vi "电机控制.vi"() -> ()   [LabVIEW 2016]
uses:
  <vilib>/Instr/_visa.llb/VISA Configure Serial Port (Instr).vi
panel:
  in  "选项卡控件":T1
  in  "PID_控制\n方式切换":bool
  in  "复位":bool
  in  "启动电机":bool
  in  "PID":cluster{"P":sgl, "I":sgl, "D":sgl} {"D" min=0 max=100 step=0.1 format="%.1f"; "I" min=0 max=100 step=0.1 format="%.1f"; "P" min=0 max=100 step=0.1 format="%.1f"}
  in  "发送目标值":bool
  in  "目标值":u32
  in  "发送PID":bool
  out "波形图表":cluster{"实际值 ":u32, "目标值":u32}(graph)
  out "串口指示灯":bool
  in  "确定按钮":bool
  in  "串口配置簇":T2={"端口"="", "波特率"=115200, "数据位"=8, "停止位"=10, "校验位"=0} {"校验位" items=["无", "奇校验", "偶校验", "Mark", "Space"]; "停止位" items=["1"=10, "2"=20]; "数据位" items=["5"=5, "6"=6, "7"=7, "8"=8]; "波特率" items=["4800"=4800, "9600"=9600, "57600"=57600, "115200"=115200]}
  out "电机转速":u32
  out "控制模\n式显示":string
  out "转速表":u32(knob) scale=0.0..230.0
  in  "转盘":u32(knob) caption="角度控制" max=360 step=20 scale=0.0..360.0
  in  "速度控制":u32(knob) max=210 step=1 scale=0.0..210.0
  out "波形图表":dbl(graph)
  out "位置控制\nPID参数":sgl[](array[numeric])
  out "速度控制\nPID":sgl[](array[numeric])
  out "指令":string
  out "16进制字符串":string
  out "接收字节数":u32
  out "error out":errorcluster
  # "电机控制调试助手"
  # "PID配置"
  # "串口配置"
  # "操作"
  # "r/min"
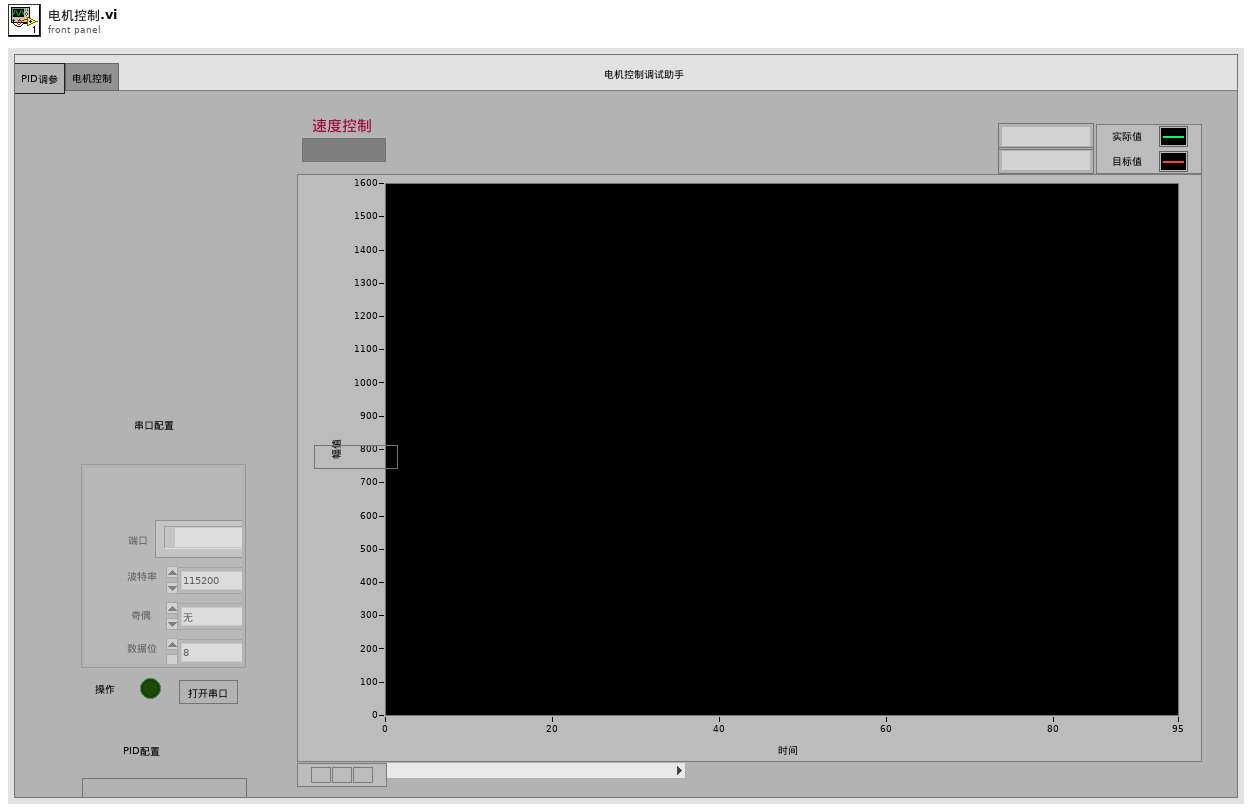
[diagram p1: front panel]
types:
  T1 = typedef "控件 2.ctl" = enum32{"PID调参", "电机控制"}
  T2 = cluster{"端口":refnum<visa-resource-name>, "波特率":u32, "数据位":u16, "停止位":u16, "校验位":u16}
  T3 = enum8{"Enabled", "Disabled", "Disabled and Grayed Out"}
  T4 = cluster{"PID[0]":sgl, "PID[1]":sgl, "PID[2]":sgl}
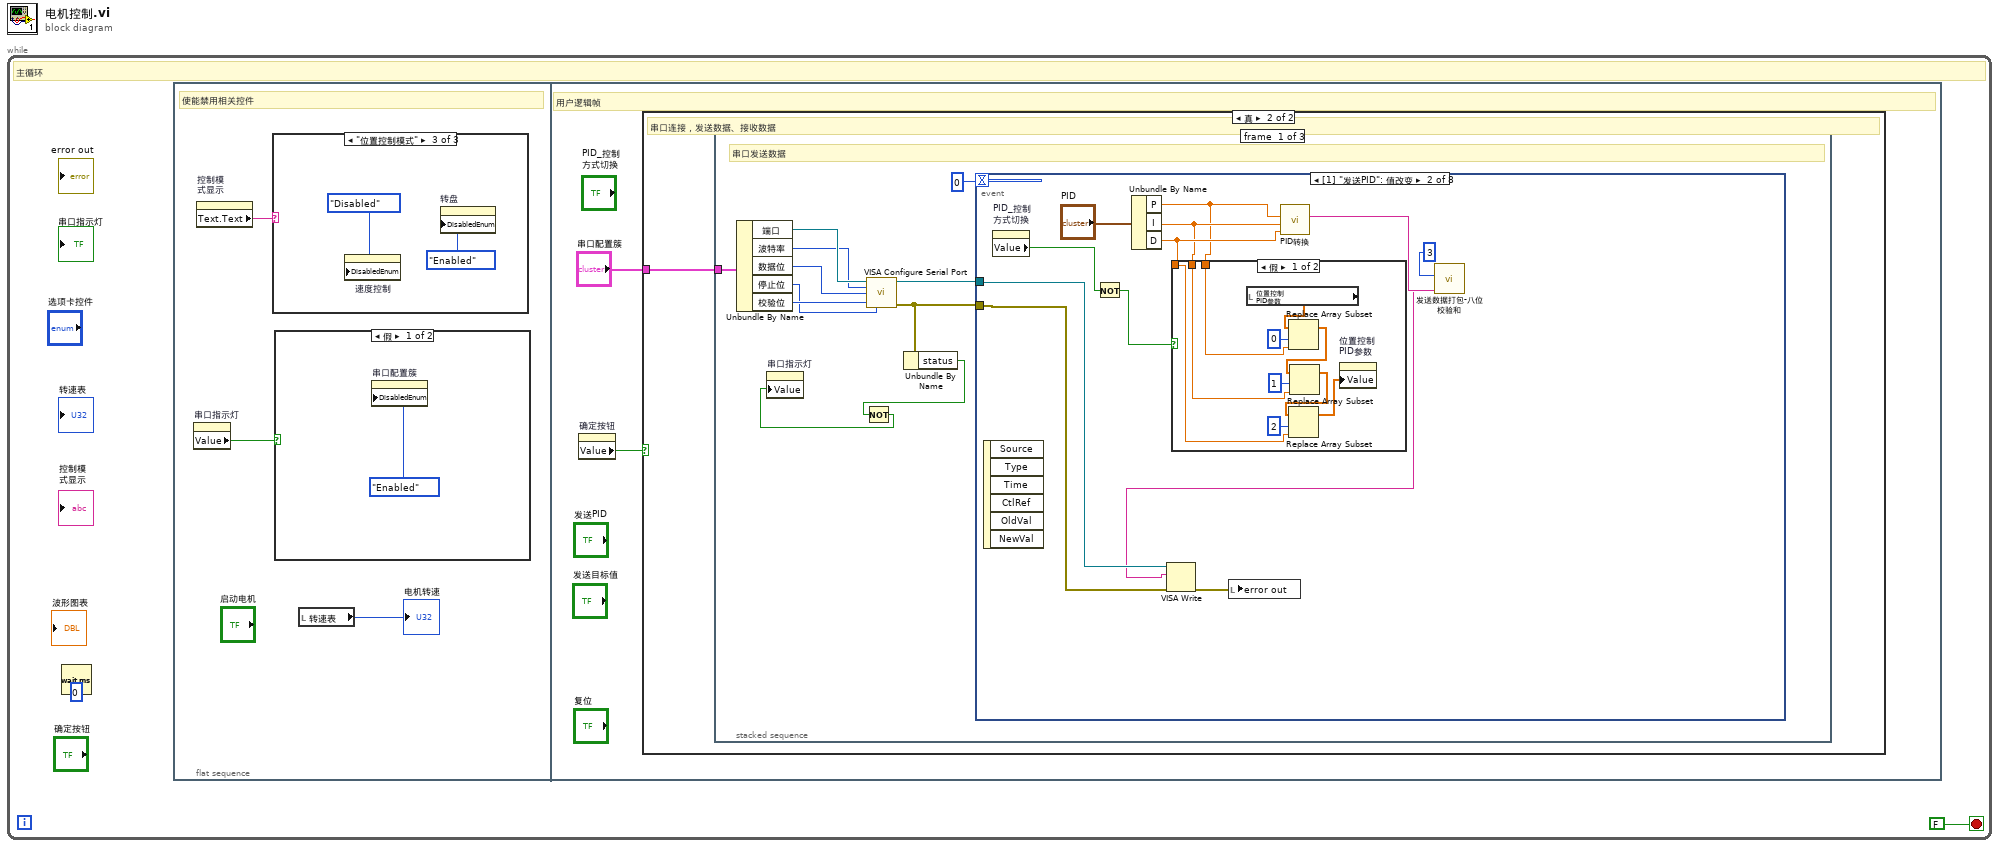
[diagram p0: block diagram]
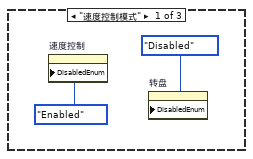
[diagram p2: hidden frame]
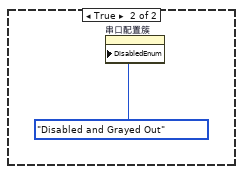
[diagram p4: hidden frame]
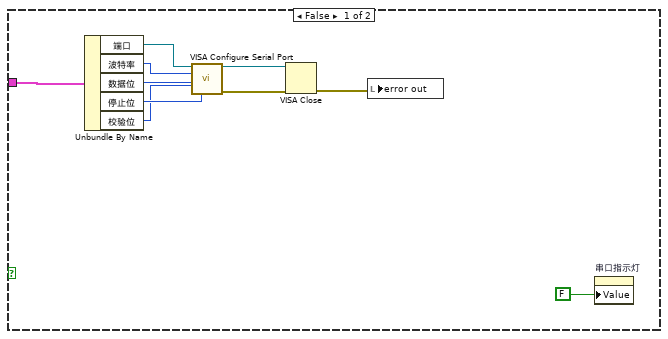
[diagram p5: hidden frame]
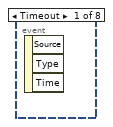
[diagram p6: hidden frame]
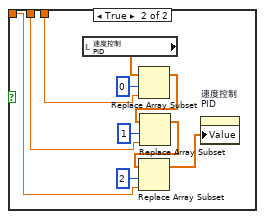
[diagram p7: hidden frame]
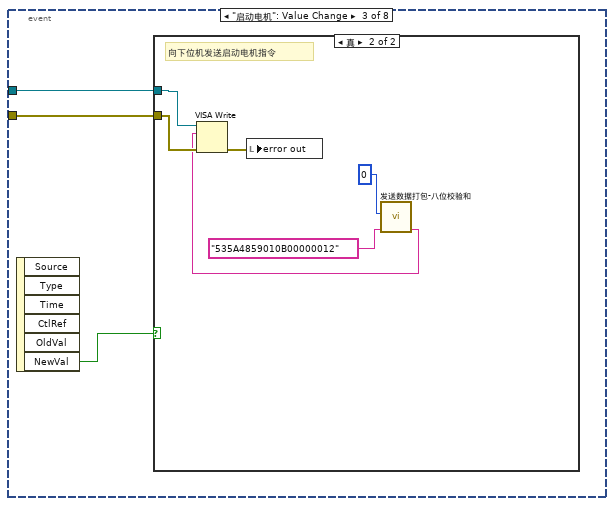
[diagram p8: hidden frame]
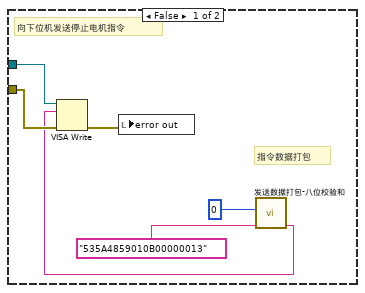
[diagram p9: hidden frame]
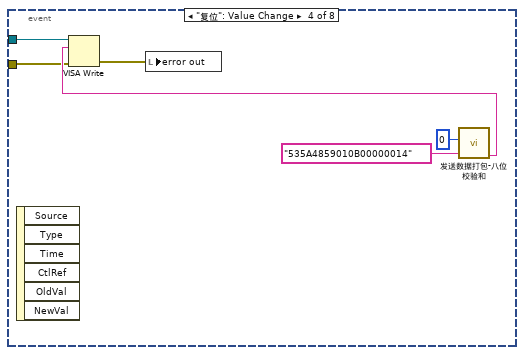
[diagram p10: hidden frame]
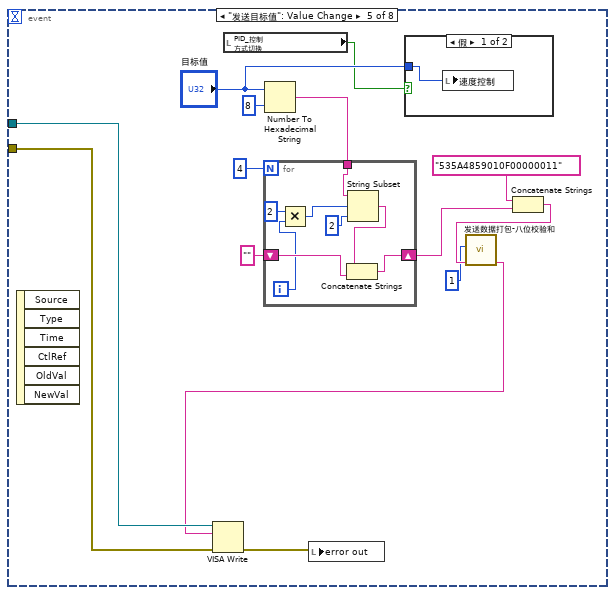
[diagram p11: hidden frame]
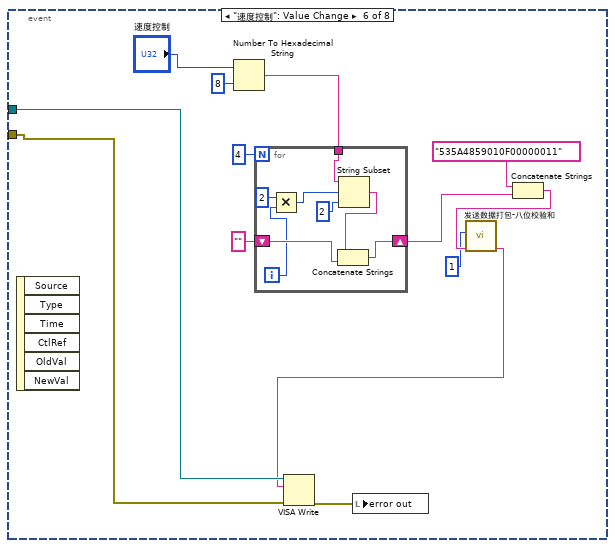
[diagram p13: hidden frame]
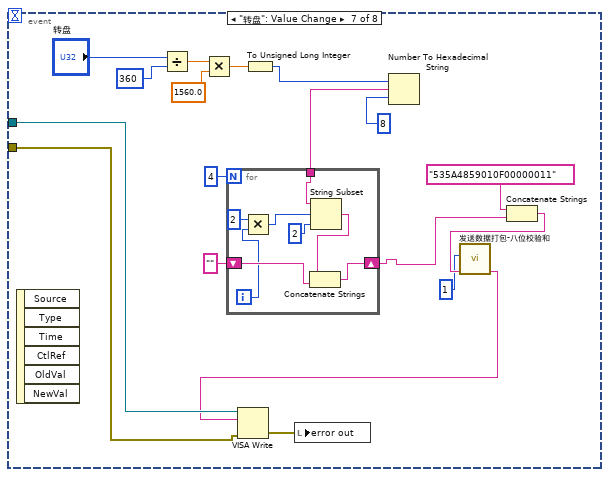
[diagram p14: hidden frame]
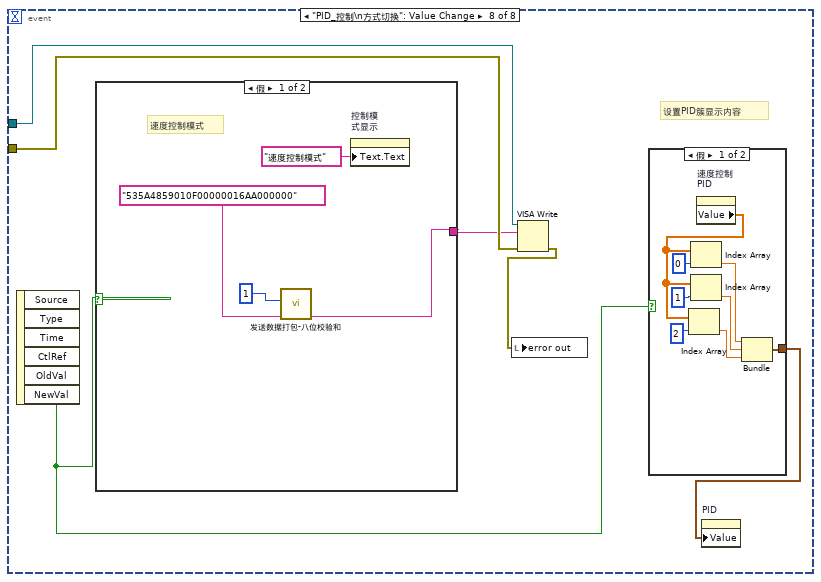
[diagram p15: hidden frame]
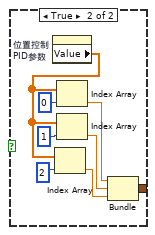
[diagram p16: hidden frame]
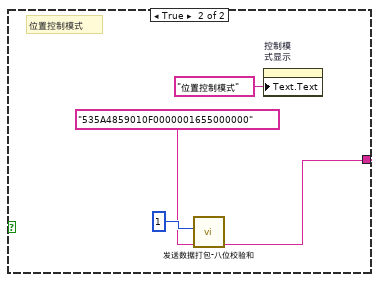
[diagram p17: hidden frame]
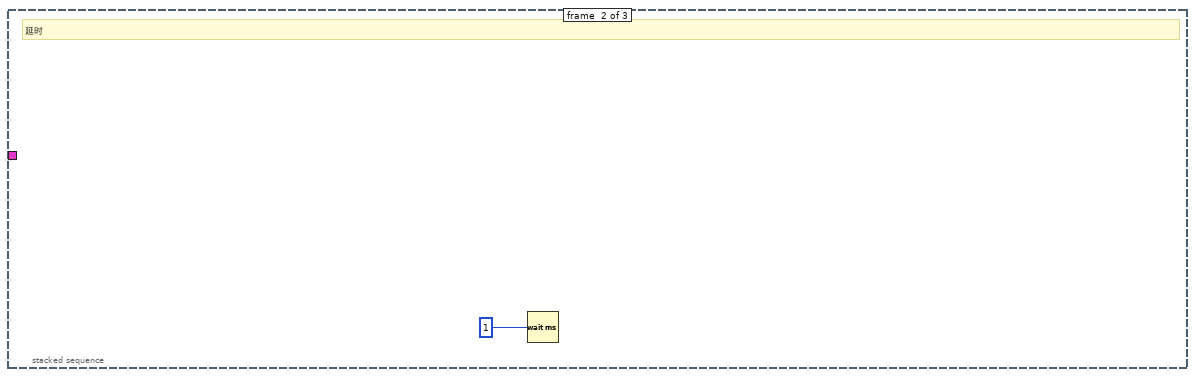
[diagram p18: hidden frame]
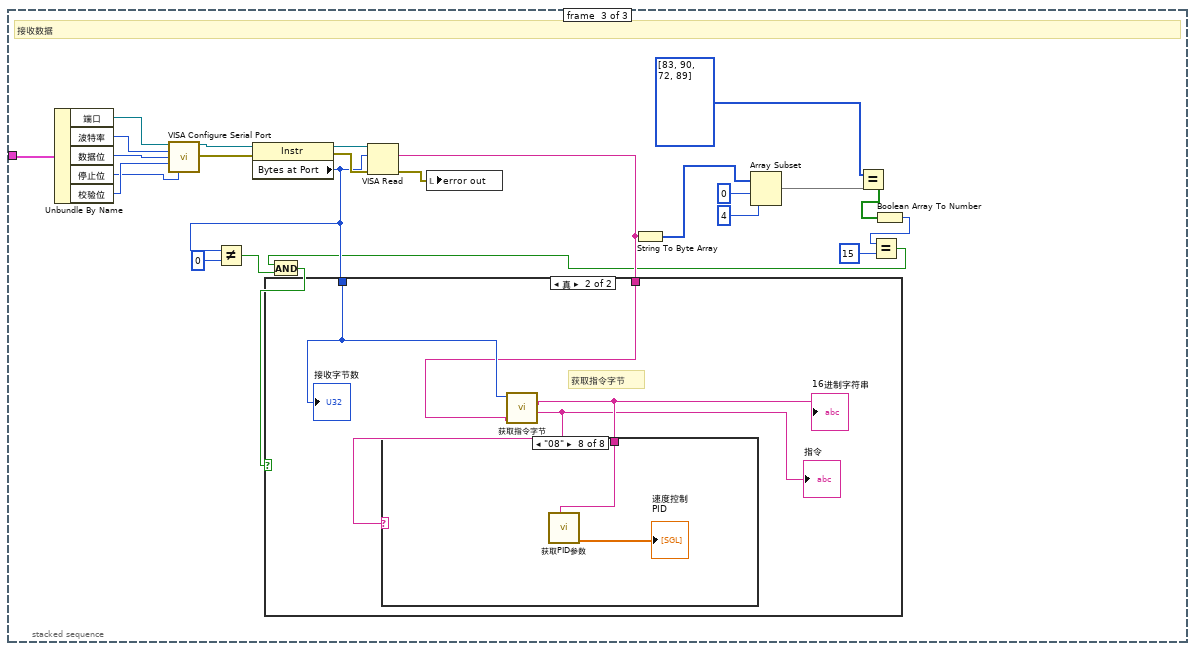
[diagram p19: hidden frame]
diagram:
  n1 = while {
    stop <- FALSE stop-if-true
    # "主循环"
    n2 = Wait (ms)(milliseconds to wait=u32 0 ("等待时间（毫秒）")) -> ()  [unwired: 1 out]
    n3 = flat-sequence {
      frame #0 {
        # "使能禁用相关控件"
        n4 = property on="串口指示灯" class="Bool (严格)"() -> ("Value"=w5:bool)  [unwired: 2 in, 2 out]
        n5 = property on="控制模\n式显示" class="Str"() -> ("Text.Text"=w3:string)  [unwired: 2 in, 2 out]
        n6 = case shown="\"位置控制模式\"" w3 {
          frame "速度控制模式" {
            n7 = property on="速度控制" class="Knob (严格)"("DisabledEnum"=T3."Enabled" ("禁用")) -> ()  [unwired: 2 in, 2 out]
            n8 = property on="转盘" class="Knob (严格)"("DisabledEnum"=T3."Disabled" ("禁用")) -> ()  [unwired: 2 in, 2 out]
          }
          frame "假", Default {
          }
          frame "位置控制模式" {
            n9 = property on="速度控制" class="Knob (严格)"("DisabledEnum"=T3."Disabled" ("禁用")) -> ()  [unwired: 2 in, 2 out]
            n10 = property on="转盘" class="Knob (严格)"("DisabledEnum"=T3."Enabled" ("禁用")) -> ()  [unwired: 2 in, 2 out]
          }
        }
        n11 = case shown="假" w5 {
          frame False {
            n12 = property on="串口配置簇" class="Clust (严格)"("DisabledEnum"=T3."Enabled" ("禁用")) -> ()  [unwired: 2 in, 2 out]
          }
          frame True {
            n13 = property on="串口配置簇" class="Clust (严格)"("DisabledEnum"=T3."Disabled and Grayed Out" ("禁用")) -> ()  [unwired: 2 in, 2 out]
          }
        }
        n14 = local read "转速表"() -> (→"电机转速":u32)
      }
      frame #1 {
        # "用户逻辑帧"
        n15 = property on="确定按钮" class="Bool (严格)"() -> ("Value"=w13:bool)  [unwired: 2 in, 2 out]
        n16 = case shown="真" w13 {
          tunnel: "串口配置簇" -> [w22 w24]
          frame False {
            n17 = Unbundle By Name(w22) -> ("端口"=w21:refnum<visa-resource-name>, "波特率"=w20:u32, "数据位"=w19:u16, "停止位"=w18:u16, "校验位"=w17:u16)
            n18 = call-poly "VISA Configure Serial Port"("VISA resource name"=w21, "baud rate (9600)"=w20, "data bits (8)"=w19, "parity (0:none)"=w17, "stop bits (10: 1 bit)"=w18) -> ("VISA resource name out"=w16:refnum<visa-resource-name>, "error out"=w15:errorcluster)  [unwired: 9 in]
            n19 = VISA Close(VISA resource name=w16, error in (no error)=w15) -> (error out=w14:errorcluster)
            n20 = local write "error out"(w14) -> ()
            n21 = property on="串口指示灯" class="Bool (严格)"("Value"=FALSE ("串口指示灯")) -> ()  [unwired: 2 in, 2 out]
          }
          frame True {
            # "串口连接，发送数据、接收数据"
            n22 = stacked-sequence {
              tunnel: w24 -> [w33 _ w214]
              frame #0 {
                # "串口发送数据"
                n23 = Unbundle By Name(w33) -> ("端口"=w32:refnum<visa-resource-name>, "波特率"=w31:u32, "数据位"=w30:u16, "停止位"=w28:u16, "校验位"=w29:u16)
                n24 = call-poly "VISA Configure Serial Port"("VISA resource name"=w32, "baud rate (9600)"=w31, "data bits (8)"=w30, "parity (0:none)"=w29, "stop bits (10: 1 bit)"=w28) -> ("VISA resource name out"=w34:refnum<visa-resource-name>, "error out"=w25:errorcluster)  [unwired: 9 in]
                n25 = Unbundle By Name(w25) -> ("status"=w27:bool)
                n26 = Not(x=w27) -> (.not. x?=w26:bool)
                n27 = property on="串口指示灯" class="Bool (严格)"("Value"=w26) -> ()  [unwired: 2 in, 2 out]
                n28 = event shown="[1] \"发送PID\": 值改变" {
                  selector: _ -> [_ _ _ _ _ _ _ _]
                  dyn-events: _ -> [_ _ _ _ _ _ _ _]
                  timeout: 0 -> [_ _ _ _ _ _ _ _]
                  tunnel: w34 -> [_ w47 w69 w84 w102 w116 w142 w164]
                  tunnel: w25 -> [_ w46 w68 w85 w101 w115 w141 w163]
                  event Timeout {
                    n29 = event-data() -> ()  [unwired: 1 in, 3 out]
                  }
                  event "发送PID": Value Change {
                    n30 = event-data() -> ()  [unwired: 1 in, 6 out]
                    n31 = property on="PID_控制\n方式切换" class="Bool (严格)"() -> ("Value"=w37:bool)  [unwired: 2 in, 2 out]
                    n32 = Not(x=w37) -> (.not. x?=w36:bool)
                    n33 = Unbundle By Name("PID") -> ("P"=w38:sgl, "I"=w39:sgl, "D"=w40:sgl)
                    n34 = case shown="假" w36 {
                      tunnel: w40 -> [w48 w59]
                      tunnel: w39 -> [w49 w60]
                      tunnel: w38 -> [w50 w61]
                      frame False {
                        n35 = local read "位置控制\nPID参数"() -> (w52:sgl[])
                        n36 = Replace Array Subset(array=w52, new element=w50, index=0 ("索引")) -> (w54:sgl[])
                        n37 = Replace Array Subset(array=w54, new element=w49, index=1 ("索引")) -> (w53:sgl[])
                        n38 = Replace Array Subset(array=w53, new element=w48, index=2 ("索引")) -> (w51:sgl[])
                        n39 = property on="位置控制\nPID参数" class="Arr (严格)"("Value"=w51) -> ()  [unwired: 2 in, 2 out]
                      }
                      frame True {
                        n40 = local read "速度控制\nPID"() -> (w67:sgl[])
                        n41 = Replace Array Subset(array=w67, new element=w61, index=0 ("索引")) -> (w66:sgl[])
                        n42 = Replace Array Subset(array=w66, new element=w60, index=1 ("索引")) -> (w65:sgl[])
                        n43 = Replace Array Subset(array=w65, new element=w59, index=2 ("索引")) -> (w58:sgl[])
                        n44 = property on="速度控制\nPID" class="Arr (严格)"("Value"=w58) -> ()  [unwired: 2 in, 2 out]
                      }
                    }
                    n45 = call "PID转换.vi"("P"=w38, "I"=w39, "D"=w40) -> ("PID"=w43:string)  [unwired: 7 in]
                    n46 = call "发送数据打包-八位校验和.vi"("16进制字符串"=w43, "命令数"=u8 3) -> ("结果字符串"=w42:string)  [unwired: 8 in, 1 out]
                    n47 = VISA Write(VISA resource name=w47, write buffer=w42, error in (no error)=w46) -> (error out=w45:errorcluster)  [unwired: 2 out]
                    n48 = local write "error out"(w45) -> ()
                  }
                  event "启动电机": Value Change {
                    n49 = event-data() -> ("NewVal"=w70:bool)  [unwired: 1 in, 5 out]
                    n50 = case shown="真" w70 {
                      tunnel: w69 -> [w73 w81]
                      tunnel: w68 -> [w72 w82]
                      frame False {
                        # "指令数据打包"
                        # "向下位机发送停止电机指令"
                        n51 = call "发送数据打包-八位校验和.vi"("16进制字符串"="535A4859010B00000013", "命令数"=u8 0) -> ("结果字符串"=w71:string)  [unwired: 8 in, 1 out]
                        n52 = VISA Write(VISA resource name=w73, write buffer=w71, error in (no error)=w72) -> (error out=w76:errorcluster)  [unwired: 2 out]
                        n53 = local write "error out"(w76) -> ()
                      }
                      frame True {
                        # "向下位机发送启动电机指令"
                        n54 = call "发送数据打包-八位校验和.vi"("16进制字符串"="535A4859010B00000012", "命令数"=u8 0) -> ("结果字符串"=w77:string)  [unwired: 8 in, 1 out]
                        n55 = VISA Write(VISA resource name=w81, write buffer=w77, error in (no error)=w82) -> (error out=w80:errorcluster)  [unwired: 2 out]
                        n56 = local write "error out"(w80) -> ()
                      }
                    }
                  }
                  event "复位": Value Change {
                    n57 = event-data() -> ()  [unwired: 1 in, 6 out]
                    n58 = call "发送数据打包-八位校验和.vi"("16进制字符串"="535A4859010B00000014", "命令数"=u8 0) -> ("结果字符串"=w86:string)  [unwired: 8 in, 1 out]
                    n59 = VISA Write(VISA resource name=w84, write buffer=w86, error in (no error)=w85) -> (error out=w83:errorcluster)  [unwired: 2 out]
                    n60 = local write "error out"(w83) -> ()
                  }
                  event "发送目标值": Value Change {
                    n61 = event-data() -> ()  [unwired: 1 in, 6 out]
                    n62 = local read "PID_控制\n方式切换"() -> (w89:bool)
                    n63 = Number To Hexadecimal String(1:i16 8 ("宽度(-)"), 2:"目标值") -> (0:w98:string)
                    n64 = for {
                      N: 4 -> [_]
                      tunnel: w98 -> [w111]
                      shift-right: [w109] -> w94
                      shift-left: "" -> [w108]
                      i -> [w106]
                      n65 = Multiply(x=2, y=w106) -> (x*y=w104:i32)
                      n66 = String Subset(string=w111, offset (0)=w104, length (rest)=u8 2 ("y")) -> (substring=w107:string)
                      n67 = Concatenate Strings(w107, w108) -> (w109:string)
                    }
                    n68 = case shown="假" w89 {
                      tunnel: "目标值" -> [w103 _]
                      frame False {
                        n69 = local write "速度控制"(w103) -> ()
                      }
                      frame True {
                      }
                    }
                    n70 = Concatenate Strings("535A4859010F00000011", w94) -> (w93:string)
                    n71 = call "发送数据打包-八位校验和.vi"("16进制字符串"=w93, "命令数"=u8 1) -> ("结果字符串"=w91:string)  [unwired: 8 in, 1 out]
                    n72 = VISA Write(VISA resource name=w102, write buffer=w91, error in (no error)=w101) -> (error out=w100:errorcluster)  [unwired: 2 out]
                    n73 = local write "error out"(w100) -> ()
                  }
                  event "速度控制": Value Change {
                    n74 = event-data() -> ()  [unwired: 1 in, 6 out]
                    n75 = Number To Hexadecimal String(1:i16 8 ("宽度(-)"), 2:"速度控制") -> (0:w123:string)
                    n76 = for {
                      N: 4 -> [_]
                      tunnel: w123 -> [w132]
                      shift-right: [w130] -> w119
                      shift-left: "" -> [w129]
                      i -> [w127]
                      n77 = Multiply(x=2, y=w127) -> (x*y=w125:i32)
                      n78 = String Subset(string=w132, offset (0)=w125, length (rest)=u8 2 ("y")) -> (substring=w128:string)
                      n79 = Concatenate Strings(w128, w129) -> (w130:string)
                    }
                    n80 = Concatenate Strings("535A4859010F00000011", w119) -> (w121:string)
                    n81 = call "发送数据打包-八位校验和.vi"("16进制字符串"=w121, "命令数"=u8 1) -> ("结果字符串"=w113:string)  [unwired: 8 in, 1 out]
                    n82 = VISA Write(VISA resource name=w116, write buffer=w113, error in (no error)=w115) -> (error out=w114:errorcluster)  [unwired: 2 out]
                    n83 = local write "error out"(w114) -> ()
                  }
                  event "转盘": Value Change {
                    n84 = event-data() -> ()  [unwired: 1 in, 6 out]
                    n85 = Divide(x="转盘", y=u32 360) -> (x/y=w136:dbl)
                    n86 = Multiply(x=w136, y=1560.0) -> (x*y=w134:dbl)
                    n87 = To Unsigned Long Integer(number=w134) -> (unsigned 32bit integer=w133:u32)
                    n88 = Number To Hexadecimal String(1:i16 8 ("宽度(-)"), 2:w133) -> (0:w149:string)
                    n89 = for {
                      N: 4 -> [_]
                      tunnel: w149 -> [w158]
                      shift-right: [w156] -> w143
                      shift-left: "" -> [w155]
                      i -> [w153]
                      n90 = Multiply(x=2, y=w153) -> (x*y=w151:i32)
                      n91 = String Subset(string=w158, offset (0)=w151, length (rest)=u8 2 ("y")) -> (substring=w154:string)
                      n92 = Concatenate Strings(w154, w155) -> (w156:string)
                    }
                    n93 = Concatenate Strings("535A4859010F00000011", w143) -> (w145:string)
                    n94 = call "发送数据打包-八位校验和.vi"("16进制字符串"=w145, "命令数"=u8 1) -> ("结果字符串"=w139:string)  [unwired: 8 in, 1 out]
                    n95 = VISA Write(VISA resource name=w142, write buffer=w139, error in (no error)=w141) -> (error out=w140:errorcluster)  [unwired: 2 out]
                    n96 = local write "error out"(w140) -> ()
                  }
                  event "PID_控制\n方式切换": Value Change {
                    # "设置PID簇显示内容"
                    n97 = event-data() -> ("NewVal"=w159:bool)  [unwired: 1 in, 5 out]
                    n98 = case shown="假" w159 {
                      tunnel: [w182 w186] -> w162
                      frame False {
                        # "速度控制模式"
                        n99 = call "发送数据打包-八位校验和.vi"("16进制字符串"="535A4859010F00000016AA000000", "命令数"=u8 1) -> ("结果字符串"=w182:string)  [unwired: 8 in, 1 out]
                        n100 = property on="控制模\n式显示" class="Str"("Text.Text"="速度控制模式" ("文本.文本")) -> ()  [unwired: 2 in, 2 out]
                      }
                      frame True {
                        # "位置控制模式"
                        n101 = call "发送数据打包-八位校验和.vi"("16进制字符串"="535A4859010F0000001655000000", "命令数"=u8 1) -> ("结果字符串"=w186:string)  [unwired: 8 in, 1 out]
                        n102 = property on="控制模\n式显示" class="Str"("Text.Text"="位置控制模式" ("文本.文本")) -> ()  [unwired: 2 in, 2 out]
                      }
                    }
                    n103 = VISA Write(VISA resource name=w164, write buffer=w162, error in (no error)=w163) -> (error out=w161:errorcluster)  [unwired: 2 out]
                    n104 = local write "error out"(w161) -> ()
                    n105 = case shown="假" w159 {
                      tunnel: [w165 w173] -> w160
                      frame False {
                        n106 = property on="速度控制\nPID" class="Arr (严格)"() -> ("Value"=w166:sgl[])  [unwired: 2 in, 2 out]
                        n107 = Index Array(array=w166, index=2 ("索引")) -> (element=w167:sgl)
                        n108 = Index Array(array=w166, index=0 ("索引")) -> (element=w170:sgl)
                        n109 = Index Array(array=w166, index=1 ("索引")) -> (element=w169:sgl)
                        n110 = Bundle(w170, w169, w167) -> (w165:cluster{sgl, sgl, sgl})  [unwired: 1 in]
                      }
                      frame True {
                        n111 = property on="位置控制\nPID参数" class="Arr (严格)"() -> ("Value"=w176:sgl[])  [unwired: 2 in, 2 out]
                        n112 = Index Array(array=w176, index=2 ("索引")) -> (element=w174:sgl)
                        n113 = Index Array(array=w176, index=0 ("索引")) -> (element=w178:sgl)
                        n114 = Index Array(array=w176, index=1 ("索引")) -> (element=w177:sgl)
                        n115 = Bundle(w178, w177, w174) -> (w173:cluster{sgl, sgl, sgl})  [unwired: 1 in]
                      }
                    }
                    n116 = property on="PID" class="Clust (严格)"("Value"=w160) -> ()  [unwired: 2 in, 2 out]
                  }
                }
              }
              frame #1 {
                # "延时"
                n117 = Wait (ms)(milliseconds to wait=u32 1 ("等待时间（毫秒）")) -> ()  [unwired: 1 out]
              }
              frame #2 {
                # "接收数据"
                n118 = Unbundle By Name(w214) -> ("端口"=w213:refnum<visa-resource-name>, "波特率"=w212:u32, "数据位"=w207:u16, "停止位"=w205:u16, "校验位"=w206:u16)
                n119 = call-poly "VISA Configure Serial Port"("VISA resource name"=w213, "baud rate (9600)"=w212, "data bits (8)"=w207, "parity (0:none)"=w206, "stop bits (10: 1 bit)"=w205) -> ("VISA resource name out"=w211:refnum<visa-resource-name>, "error out"=w210:errorcluster)  [unwired: 9 in]
                n120 = property class="Instr"(reference=w211, error in=w210) -> (reference out=w209:refnum<visa-resource-name>, error out=w208:errorcluster, "Bytes at Port"=w203:u32)
                n121 = Not Equal?(x=w203, y=u32 0) -> (x != y?=w193:bool)
                n122 = VISA Read(VISA resource name=w209, byte count=w203, error in (no error)=w208) -> (read buffer=w196:string, error out=w202:errorcluster)  [unwired: 2 out]
                n123 = local write "error out"(w202) -> ()
                n124 = String To Byte Array(string=w196) -> (unsigned byte array=w190:u8[])
                n125 = Array Subset(array=w190, index=0 ("索引"), length=4 ("长度")) -> (w198:u8[])
                n126 = Equal?(x=u8[] [83, 90, 72, 89], y=w198) -> (x = y?=w199:bool[])
                n127 = Boolean Array To Number(Boolean array=w199) -> (number=w195:u32)
                n128 = Equal?(x=w195, y=u32 15) -> (x = y?=w192:bool)
                n129 = And(x=w192, y=w193) -> (x .and. y?=w191:bool)
                n130 = case shown="真" w191 {
                  tunnel: w196 -> [_ w217]
                  tunnel: w203 -> [_ w218]
                  frame False {
                  }
                  frame True {
                    # "获取指令字节"
                    n131 = call "获取指令字节.vi"("字符串"=w217, "字节数"=w218) -> ("指令"=w215:string, "16进制字符串"=w216:string)  [unwired: 8 in]
                    "16进制字符串" <- w216
                    "指令" <- w215
                    n132 = case shown="\"08\"" w215 {
                      tunnel: w216 -> [_ w221 w226 w231 _ _ w237 w241]
                      frame "假", Default {
                      }
                      frame "01" {
                        n133 = call "获取实际值.vi"("字符串"=w221) -> ("实际值字符串"=w220:string)  [unwired: 9 in, 1 out]
                        n134 = Hexadecimal String To Number(string=w220) -> (number=w219:u32)  [unwired: 2 in, 1 out]
                        n135 = property on="目标值" class="DigNum (严格)"("Value"=w219) -> ()  [unwired: 2 in, 2 out]
                      }
                      frame "02" {
                        # "获取实际值"
                        # "下位机发送实际值"
                        n136 = local read "目标值"() -> (w225:u32)
                        n137 = call "获取实际值.vi"("字符串"=w226) -> ("实际值"=w222:u32)  [unwired: 9 in, 1 out]
                        n138 = local read "PID_控制\n方式切换"() -> (w223:bool)
                        n139 = Bundle("实际值"=w222, "目标值"=w225) -> (→"波形图表":cluster{"实际值 ":u32, "目标值":u32})  [unwired: 1 in]
                        n140 = case shown="假" w223 {
                          tunnel: w222 -> [w227 w228]
                          frame False {
                            n141 = local write "转速表"(w227) -> ()
                            n142 = local write "波形图表"(w227) -> ()
                          }
                          frame True {
                            n143 = local write "波形图表"(w228) -> ()
                          }
                        }
                      }
                      frame "03" {
                        # "获取PID参数"
                        n144 = call "获取PID参数.vi"("字符串"=w231) -> ("PID"=w230:sgl[])  [unwired: 10 in]
                        "位置控制\nPID参数" <- w230
                        n145 = Array To Cluster(array=w230) -> (cluster=w229:T4)
                        n146 = local write "PID"(w229) -> ()
                      }
                      frame "04" {
                        # "下位机发送启动按钮状态"
                        n147 = property on="启动电机" class="Bool (严格)"("Value"=TRUE ("启动电机")) -> ()  [unwired: 2 in, 2 out]
                      }
                      frame "05" {
                        # "下位机发送停止按钮状态"
                        n148 = property on="启动电机" class="Bool (严格)"("Value"=FALSE ("启动电机")) -> ()  [unwired: 2 in, 2 out]
                      }
                      frame "07" {
                        n149 = call "获取实际值.vi"("字符串"=w237) -> ("实际值字符串"=w236:string)  [unwired: 9 in, 1 out]
                        n150 = Equal?(x="00000055", y=w236) -> (x = y?=w234:bool)
                        n151 = case shown="假" w234 {
                          frame False {
                            n152 = property on="PID_控制\n方式切换" class="Bool (严格)"("Value"=FALSE ("控制方式切换")) -> ()  [unwired: 2 in, 2 out]
                          }
                          frame True {
                            n153 = property on="PID_控制\n方式切换" class="Bool (严格)"("Value"=TRUE ("控制方式切换")) -> ()  [unwired: 2 in, 2 out]
                          }
                        }
                      }
                      frame "08" {
                        n154 = call "获取PID参数.vi"("字符串"=w241) -> ("PID"=→"速度控制\nPID":sgl[])  [unwired: 10 in]
                      }
                    }
                    "接收字节数" <- w218
                  }
                }
              }
            }
          }
        }
      }
    }
  }
